vi "BlinkM GetRGB.vi"(0 "Arduino Resource":T1={"VISA resource"="", "Board Type"=enum."Uno", "Connection Type"=enum."USB / Serial", "Bytes Per Packet (15)"=15}, 7 "Address":u8, 11 "error in":errorcluster) -> (4 "Arduino Resource":T1={"VISA resource"="", "Board Type"=enum."Uno", "Connection Type"=enum."USB / Serial", "Bytes Per Packet (15)"=15}, 8 "Color":u32(colorbox), 15 "error out":errorcluster)   [LabVIEW 2015, in "LabVIEW Interface for Arduino.lvlib"]
doc: "Get the current RGB color of the specified BlinkM."
uses:
  <vilib>/LabVIEW Interface for Arduino/LabVIEW Interface for Arduino.lvlib
  <vilib>/LabVIEW Interface for Arduino/Type Defs/Arduino Resource.ctl
  <vilib>/LabVIEW Interface for Arduino/Type Defs/Board Type.ctl
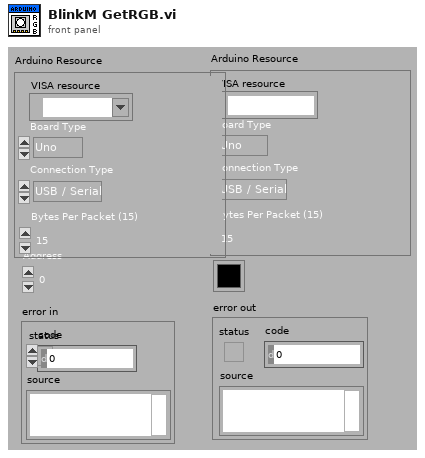
[diagram p1: front panel]
types:
  T1 = typedef "LabVIEW Interface for Arduino.lvlib/Arduino Resource.ctl" = cluster{"VISA resource":refnum<visa-resource-name>, "Board Type":T2, "Connection Type":enum8{"USB / Serial"}, "Bytes Per Packet (15)":u8}
  T2 = typedef "LabVIEW Interface for Arduino.lvlib/Board Type.ctl" = enum16{"Uno", "Dimuelanove w/Atmega 328", "Mega 2560"}
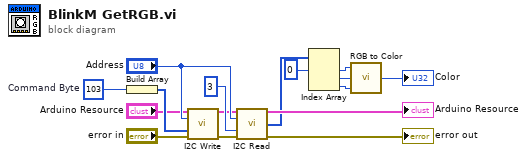
[diagram p0: block diagram]
diagram:
  w15 = u8 103  # Command Byte
  n1 = Build Array(w15) -> (w14:u8[])
  n2 = call <vilib>:"I2C Write.vi"("Arduino Resource"="Arduino Resource", "Address (0)"="Address", "I2C Data Bytes"=w14, "error in"="error in") -> ("Arduino Resource"=w3:T1, "error out"=w13:errorcluster)  [unwired: 10 in]
  n3 = call <vilib>:"I2C Read.vi"("Arduino Resource"=w3, "Address (0)"="Address", "Bytes To Read"=u8 3, "error in"=w13) -> ("Arduino Resource"=→"Arduino Resource":T1, "I2C Data"=w1:u8[], "error out"=→"error out":errorcluster)  [unwired: 9 in]
  n4 = Index Array(array=w1, index #1=0 ("index")) -> (element #1=w8:u8, element #2=w7:u8, element #3=w6:u8)  [unwired: 2 in]
  n5 = call <vilib>:"RGB to Color.vi"("B"=w6, "G"=w7, "R"=w8) -> ("Color"=→"Color":u32)
